vi "Configure Multipoint.vi"(7 "Output Mode (0: Fixed)":u16(ring) items=["Fixed", "Sweep", "List"], 8 "error in (no error)":errorcluster, 9 "Trigger Count (1)":i32=1 format="%#.6g", 10 "Number of Times to Arm (1)":i32=1 format="%#.6g", 11 "VISA resource name":refnum<visa-resource-name>) -> (0 "error out":errorcluster, 3 "VISA resource name out":refnum<visa-resource-name>)   [LabVIEW 2010, in "Keithley 24XX.lvlib"]
doc: "Configures trigger count and sample count so you can take multipoint measurements.\n\n<B>Note</B> Use this VI only with other low-level VIs. The high-level VIs automatically incorporate this functionality. This VI does not check the instrument status. If you want to check the instrument status, call the Error Query VI at the conclusion of the sequence."
uses:
  <instrlib>/Keithley 24XX/Keithley 24XX.lvlib
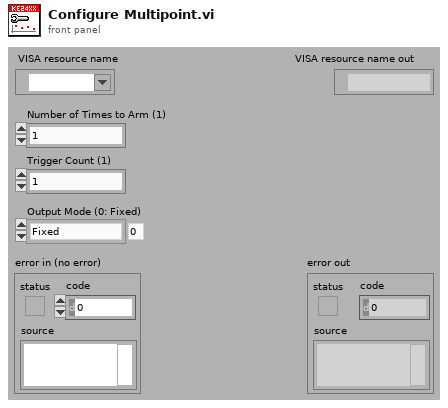
[diagram p1: front panel]
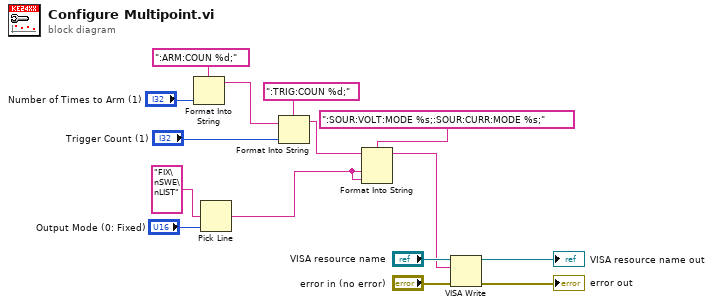
[diagram p0: block diagram]
diagram:
  n1 = Format Into String(format string=":ARM:COUN %d;", "Number of Times to Arm (1)") -> (resulting string=w9:string)  [unwired: 2 in, 1 out]
  n2 = Pick Line(multi-line string="FIX\nSWE\nLIST", line index="Output Mode (0: Fixed)") -> (output string=w3:string)  [unwired: 1 in]
  n3 = Format Into String(format string=":TRIG:COUN %d;", initial string=w9, "Trigger Count (1)") -> (resulting string=w8:string)  [unwired: 1 in, 1 out]
  n4 = Format Into String(format string=":SOUR:VOLT:MODE %s;:SOUR:CURR:MODE %s;", initial string=w8, w3, w3) -> (resulting string=w7:string)  [unwired: 1 in, 1 out]
  n5 = VISA Write(VISA resource name="VISA resource name", write buffer=w7, error in (no error)="error in (no error)") -> (VISA resource name out=→"VISA resource name out":refnum<visa-resource-name>, error out=→"error out":errorcluster)  [unwired: 1 out]
